vi "Registry.vi"(11 "registry actions":refnum<user-event>) -> ()   [LabVIEW 2018, in "GLog.lvlib" / "Registry.lvlib"]
uses:
  Registry.lvlib
  Registry Message.ctl
  Registry Actions.ctl
  api/logger_class/Logger.lvclass
  <vilib>/event_ctls.llb/usereventprio.ctl
  api/logger_class/Logger.lvclass/Logger.ctl
  api/Log Record.ctl
  api/logger_class/Internal Log Levels.ctl
  <vilib>/Utility/error.llb/Error Cluster From Error Code.vi
  api/logger_class/Log (Log Record).vi
  <vilib>/ErrorRing/Error Ring.xnode
  reuse_library/Utilities/Utilities.lvlib
  api/GLog.lvlib
panel:
  # "Connector Pane"
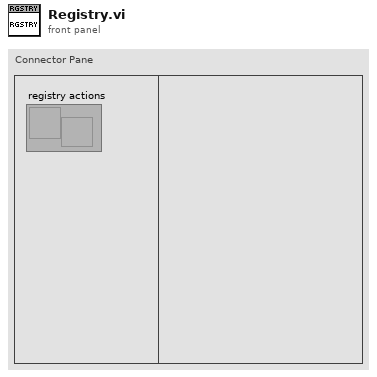
[diagram p1: front panel]
types:
  T1 = typedef "usereventprio.ctl" = enum32{"high priority", "normal priority"}
  T2 = typedef "GLog.lvlib/Registry.lvlib/Registry Message.ctl" = cluster{"action":T3, "data":variant, "return notifier":refnum<notifier>}
  T3 = typedef "GLog.lvlib/Registry.lvlib/Registry Actions.ctl" = enum16{"Register", "Log", "Enable", "Enable All", "Disable", "Disable All", "List", "Unregister", "Unregister All", "Shutdown"}
  T4 = typedef "GLog.lvlib/Log Record.ctl" = cluster{"level":T5, "timestamp":timestamp, "call chain":string[], "message":string, "data":variant}
  T5 = typedef "GLog.lvlib/Internal Log Levels.ctl" = enum16{"Trace", "Debug", "Info", "Warning", "Error", "Critical", "Internal"}
  T6 = cluster{"logger out":refnum<class "Logger.lvclass">, "empty?":bool, "error out":errorcluster}
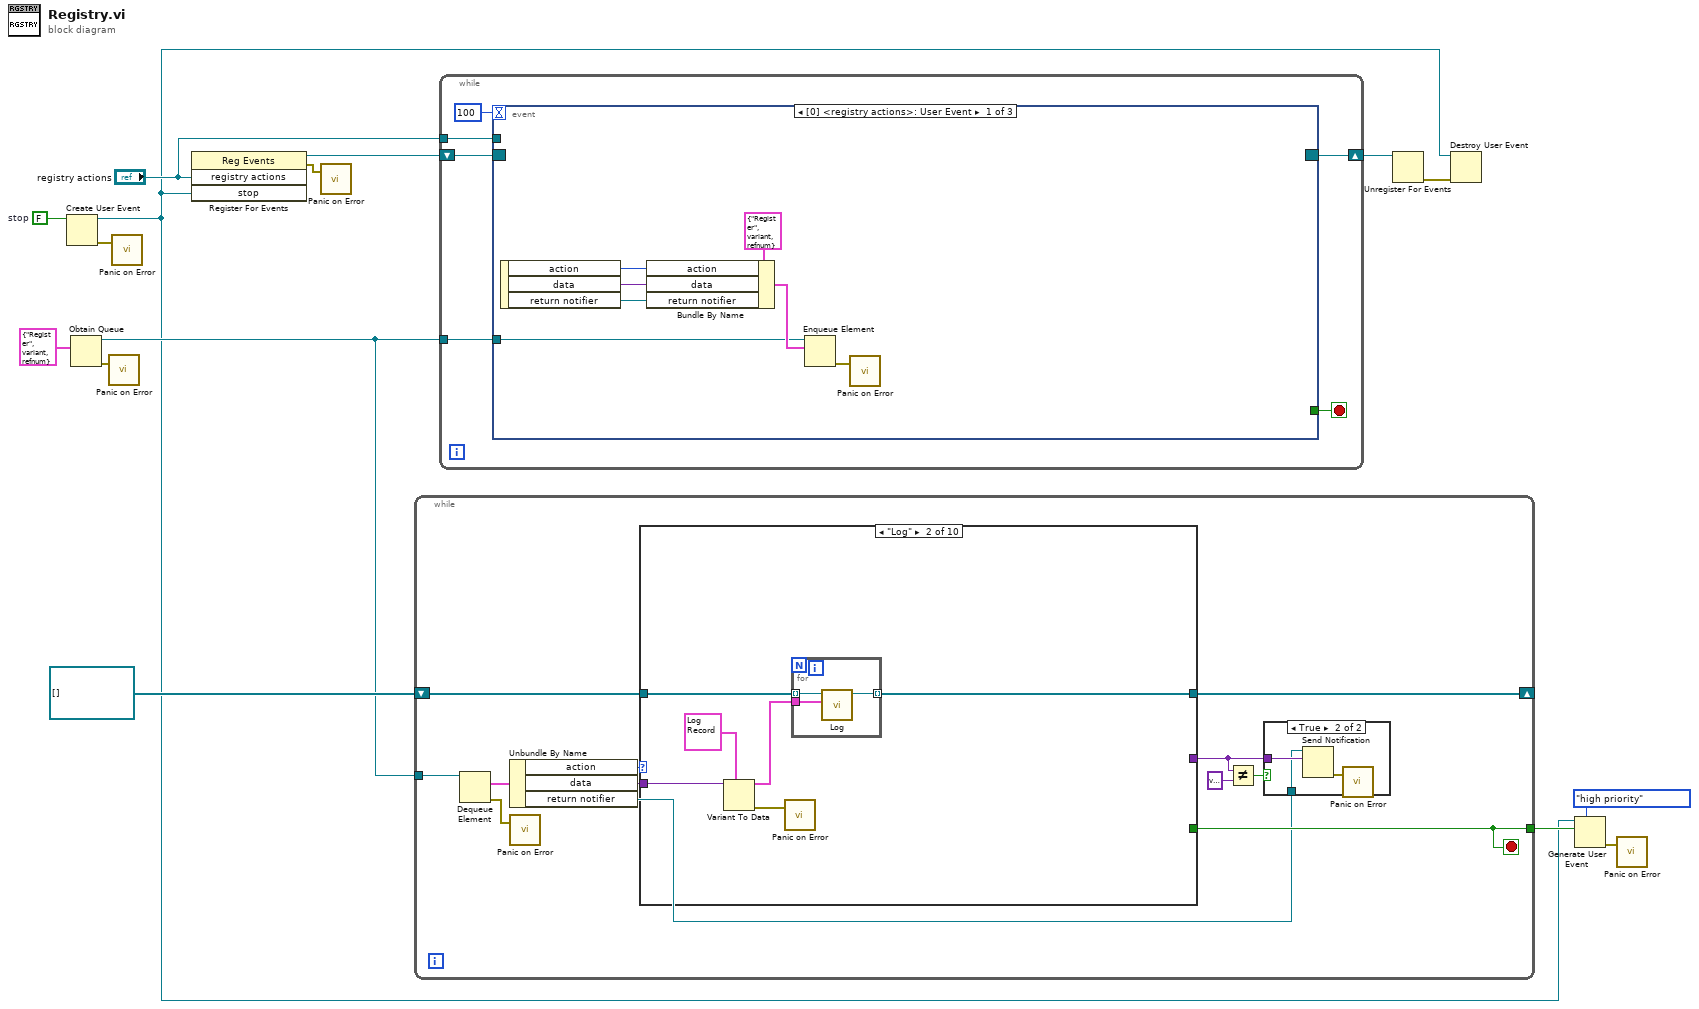
[diagram p0: block diagram]
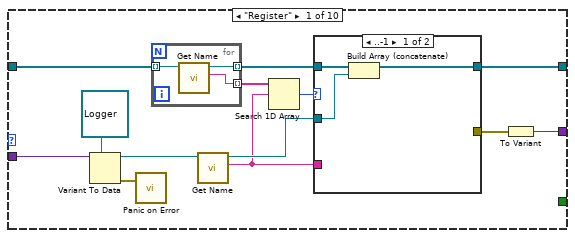
[diagram p3: hidden frame]
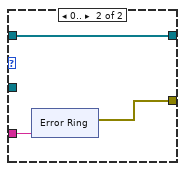
[diagram p4: hidden frame]
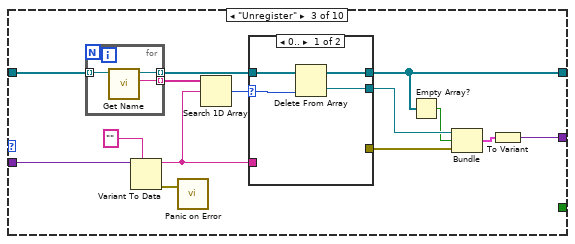
[diagram p5: hidden frame]
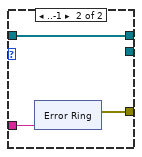
[diagram p6: hidden frame]
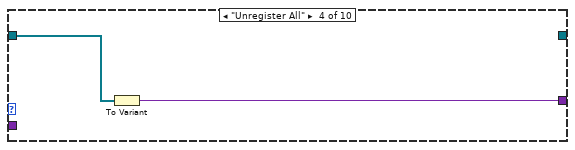
[diagram p7: hidden frame]
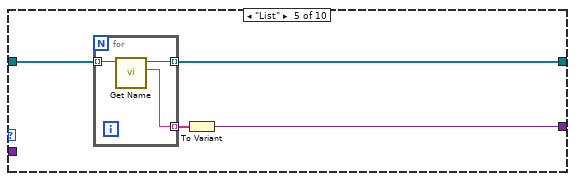
[diagram p8: hidden frame]
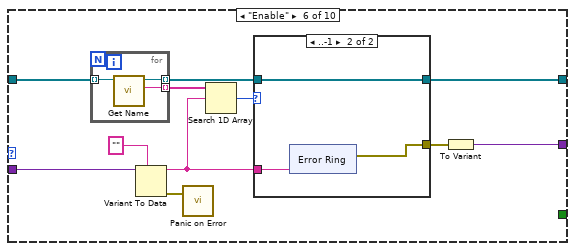
[diagram p9: hidden frame]
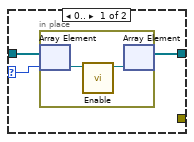
[diagram p10: hidden frame]
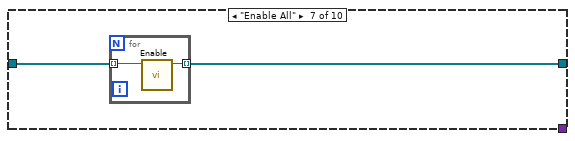
[diagram p11: hidden frame]
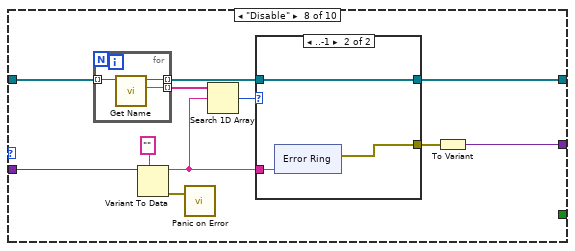
[diagram p12: hidden frame]
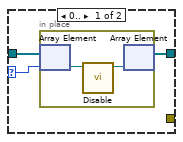
[diagram p13: hidden frame]
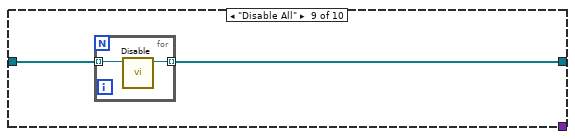
[diagram p14: hidden frame]
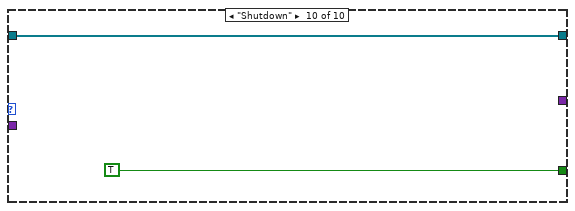
[diagram p15: hidden frame]
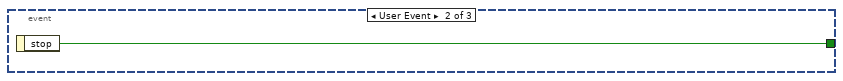
[diagram p16: hidden frame]
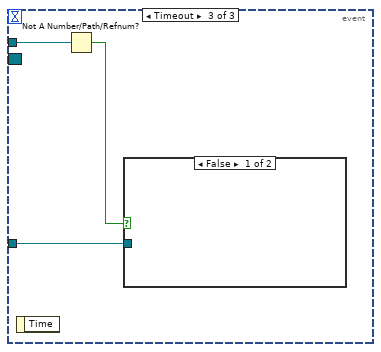
[diagram p17: hidden frame]
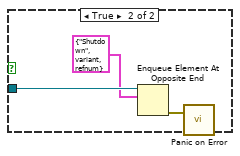
[diagram p18: hidden frame]
diagram:
  w7 = FALSE  # stop
  n1 = Create User Event(user event datatype=w7) -> (user event=w1:refnum<user-event>, error out=w6:errorcluster)  [unwired: 1 in]
  n2 = Obtain Queue(element data type=T2 {"action"=enum."Register", "data"=variant, "return notifier"=refnum} ("registry message")) -> (queue out=w13:refnum<queue>, error out=w9:errorcluster)  [unwired: 4 in, 1 out]
  n3 = call "Panic on Error.vi"("error in (no error)"=w9) -> ()  [unwired: 3 in]
  n4 = call "Panic on Error.vi"("error in (no error)"=w6) -> ()  [unwired: 3 in]
  n5 = register-events("registry actions", w1) -> (reference out=w11:refnum<event-registration>, error out=w8:errorcluster)  [unwired: 2 in]
  n6 = call "Panic on Error.vi"("error in (no error)"=w8) -> ()  [unwired: 3 in]
  n7 = while {
    shift-right: [w27] -> _
    shift-left: refnum<class "Logger.lvclass">[] [] -> [w26]
    tunnel: w13 -> [w25]
    tunnel: [w20] -> w5
    stop <- w20 stop-if-true
    n8 = Dequeue Element(queue=w25) -> (element=w23:T2, error out=w21:errorcluster)  [unwired: 2 in, 2 out]
    n9 = Unbundle By Name(w23) -> ("action"=w24:T3, "data"=w22:variant, "return notifier"=w17:refnum<notifier>)
    n10 = call "Panic on Error.vi"("error in (no error)"=w21) -> ()  [unwired: 3 in]
    n11 = case shown="\"Log\"" w24 {
      tunnel: w22 -> [w43 w64 w81 _ _ w111 _ w145 _ _]
      tunnel: [w41 w62 w70 _ w104 w112 w138 w144 w171 w176] -> w27
      tunnel: w26 -> [w39 w65 w82 w101 w105 w113 w139 w146 w172 w176]
      tunnel: [w31 _ w71 w100 w102 w109 _ w142 _ _] -> w16
      tunnel: [_ _ _ _ _ _ _ _ _ TRUE] -> w20
      frame "Register" {
        n12 = Variant To Data(type=refnum<class "Logger.lvclass"> refnum ("Logging.lvlib:Logger.lvclass"), Variant=w43) -> (data=w37:refnum<class "Logger.lvclass">, error out=w33:errorcluster)  [unwired: 1 in]
        n13 = call "Panic on Error.vi"("error in (no error)"=w33) -> ()  [unwired: 3 in]
        n14 = for {
          tunnel: w39 -> [w59] mode=indexing
          tunnel: [w58] -> w40 mode=indexing
          tunnel: [w57] -> w38 mode=indexing
          n15 = call "Get Name.vi"("logger in"=w59) -> ("name"=w57:string, "logger out"=w58:refnum<class "Logger.lvclass">)  [unwired: 9 in]
        }
        n16 = call "Get Name.vi"("logger in"=w37) -> ("name"=w34:string, "logger out"=w36:refnum<class "Logger.lvclass">)  [unwired: 9 in]
        n17 = Search 1D Array(1D array=w38, element=w34) -> (index of element=w35:i32)  [unwired: 1 in]
        n18 = case shown="..-1" w35 {
          tunnel: [w46 w49] -> w41
          tunnel: w40 -> [w45 w49]
          tunnel: w36 -> [w44 _]
          tunnel: w34 -> [_ w48]
          tunnel: [_ w47] -> w32
          frame ..-1 {
            n19 = Build Array (concatenate)(w45, w44) -> (w46:refnum<class "Logger.lvclass">[])
          }
          frame 0.. {
            n20 = xnode "Error Ring"("parameter 0"=w48) -> ("error out"=w47:errorcluster)
          }
        }
        n21 = To Variant(anything=w32) -> (Variant=w31:variant)
      }
      frame "Log" {
        n22 = Variant To Data(type=T4 {"level"=enum."Trace", "timestamp"=timestamp(0 s since 1904-01-01), "call chain"=[], "message"="", "data"=variant} ("log record"), Variant=w64) -> (data=w63:T4, error out=w61:errorcluster)  [unwired: 1 in]
        n23 = call "Panic on Error.vi"("error in (no error)"=w61) -> ()  [unwired: 3 in]
        n24 = for {
          tunnel: w65 -> [w68] mode=indexing
          tunnel: w63 -> [w66]
          tunnel: [w67] -> w62 mode=indexing
          n25 = call-poly "Log.vi"("log record"=w66, "Logger in"=w68) -> ("Logger out"=w67:refnum<class "Logger.lvclass">)  [unwired: 9 in]
        }
      }
      frame "Unregister" {
        n26 = for {
          tunnel: w82 -> [w99] mode=indexing
          tunnel: [w98] -> w79 mode=indexing
          tunnel: [w97] -> w77 mode=indexing
          n27 = call "Get Name.vi"("logger in"=w99) -> ("name"=w98:string, "logger out"=w97:refnum<class "Logger.lvclass">)  [unwired: 9 in]
        }
        n28 = Variant To Data(type="", Variant=w81) -> (data=w76:string, error out=w75:errorcluster)  [unwired: 1 in]
        n29 = call "Panic on Error.vi"("error in (no error)"=w75) -> ()  [unwired: 3 in]
        n30 = Search 1D Array(1D array=w79, element=w76) -> (index of element=w78:i32)  [unwired: 1 in]
        n31 = case shown="0.." w78 {
          selector: w78 -> [w85 _]
          tunnel: w77 -> [w86 w89]
          tunnel: [w84 w89] -> w70
          tunnel: w76 -> [_ w88]
          tunnel: [w83 _] -> w73
          tunnel: [_ w87] -> w74
          frame 0.. {
            n32 = Delete From Array(array=w86, index=w85) -> (deleted portion=w83:refnum<class "Logger.lvclass">, array with subset deleted=w84:refnum<class "Logger.lvclass">[])  [unwired: 1 in]
          }
          frame ..-1 {
            n33 = xnode "Error Ring"("parameter 0"=w88) -> ("error out"=w87:errorcluster)
          }
        }
        n34 = Empty Array?(array=w70) -> (empty?=w69:bool)
        n35 = Bundle("logger out"=w73, "empty?"=w69, "error out"=w74) -> (w72:T6)  [unwired: 1 in]
        n36 = To Variant(anything=w72) -> (Variant=w71:variant)
      }
      frame "Unregister All" {
        n37 = To Variant(anything=w101) -> (Variant=w100:variant)
      }
      frame "List" {
        n38 = for {
          tunnel: w105 -> [w108] mode=indexing
          tunnel: [w107] -> w104 mode=indexing
          tunnel: [w106] -> w103 mode=indexing
          n39 = call "Get Name.vi"("logger in"=w108) -> ("name"=w106:string, "logger out"=w107:refnum<class "Logger.lvclass">)  [unwired: 9 in]
        }
        n40 = To Variant(anything=w103) -> (Variant=w102:variant)
      }
      frame "Enable" {
        n41 = for {
          tunnel: w113 -> [w137] mode=indexing
          tunnel: [w136] -> w118 mode=indexing
          tunnel: [w135] -> w116 mode=indexing
          n42 = call "Get Name.vi"("logger in"=w137) -> ("name"=w136:string, "logger out"=w135:refnum<class "Logger.lvclass">)  [unwired: 9 in]
        }
        n43 = Variant To Data(type="", Variant=w111) -> (data=w115:string, error out=w114:errorcluster)  [unwired: 1 in]
        n44 = call "Panic on Error.vi"("error in (no error)"=w114) -> ()  [unwired: 3 in]
        n45 = Search 1D Array(1D array=w118, element=w115) -> (index of element=w117:i32)  [unwired: 1 in]
        n46 = case shown="..-1" w117 {
          selector: w117 -> [w121 _]
          tunnel: w116 -> [w122 w127]
          tunnel: [w120 w127] -> w112
          tunnel: w115 -> [_ w126]
          tunnel: [_ w125] -> w110
          frame 0.. {
            n47 = in-place {
              n48 = in-place-array #1(w122, w121) -> (w124:refnum<class "Logger.lvclass">)
              n49 = call "Enable.vi"("logger in"=w124) -> ("logger out"=w123:refnum<class "Logger.lvclass">)  [unwired: 10 in]
              n50 = in-place-array #1(w123) -> (w120:refnum<class "Logger.lvclass">[])  [unwired: 1 out]
            }
          }
          frame ..-1 {
            n51 = xnode "Error Ring"("parameter 0"=w126) -> ("error out"=w125:errorcluster)
          }
        }
        n52 = To Variant(anything=w110) -> (Variant=w109:variant)
      }
      frame "Enable All" {
        n53 = for {
          tunnel: w139 -> [w141] mode=indexing
          tunnel: [w140] -> w138 mode=indexing
          n54 = call "Enable.vi"("logger in"=w141) -> ("logger out"=w140:refnum<class "Logger.lvclass">)  [unwired: 10 in]
        }
      }
      frame "Disable" {
        n55 = for {
          tunnel: w146 -> [w170] mode=indexing
          tunnel: [w169] -> w151 mode=indexing
          tunnel: [w168] -> w149 mode=indexing
          n56 = call "Get Name.vi"("logger in"=w170) -> ("name"=w169:string, "logger out"=w168:refnum<class "Logger.lvclass">)  [unwired: 9 in]
        }
        n57 = Variant To Data(type="", Variant=w145) -> (data=w148:string, error out=w147:errorcluster)  [unwired: 1 in]
        n58 = call "Panic on Error.vi"("error in (no error)"=w147) -> ()  [unwired: 3 in]
        n59 = Search 1D Array(1D array=w151, element=w148) -> (index of element=w150:i32)  [unwired: 1 in]
        n60 = case shown="..-1" w150 {
          selector: w150 -> [w154 _]
          tunnel: w149 -> [w155 w160]
          tunnel: [w153 w160] -> w144
          tunnel: w148 -> [_ w159]
          tunnel: [_ w158] -> w143
          frame 0.. {
            n61 = in-place {
              n62 = in-place-array #2(w155, w154) -> (w157:refnum<class "Logger.lvclass">)
              n63 = call "Disable.vi"("logger in"=w157) -> ("logger out"=w156:refnum<class "Logger.lvclass">)  [unwired: 10 in]
              n64 = in-place-array #2(w156) -> (w153:refnum<class "Logger.lvclass">[])  [unwired: 1 out]
            }
          }
          frame ..-1 {
            n65 = xnode "Error Ring"("parameter 0"=w159) -> ("error out"=w158:errorcluster)
          }
        }
        n66 = To Variant(anything=w143) -> (Variant=w142:variant)
      }
      frame "Disable All" {
        n67 = for {
          tunnel: w172 -> [w174] mode=indexing
          tunnel: [w173] -> w171 mode=indexing
          n68 = call "Disable.vi"("logger in"=w174) -> ("logger out"=w173:refnum<class "Logger.lvclass">)  [unwired: 10 in]
        }
      }
      frame "Shutdown" {
      }
    }
    n69 = Not Equal?(x=w16, y=variant) -> (x != y?=w18:bool)
    n70 = case shown="True" w18 {
      tunnel: w17 -> [_ w29]
      tunnel: w16 -> [_ w30]
      frame False {
      }
      frame True {
        n71 = Send Notification(notification=w30, notifier=w29) -> (error out=w28:errorcluster)  [unwired: 1 in, 1 out]
        n72 = call "Panic on Error.vi"("error in (no error)"=w28) -> ()  [unwired: 3 in]
      }
    }
  }
  n73 = while {
    tunnel: w13 -> [w182]
    shift-right: [w180] -> w12
    shift-left: w11 -> [w179]
    tunnel: "registry actions" -> [w178]
    stop <- w177 stop-if-true
    n74 = event shown="[0] <registry actions>: User Event" {
      selector: w179 -> [_ _ _]
      dyn-events: [_ _ _] -> w180
      timeout: 100 -> [_ _ _]
      tunnel: w182 -> [w185 _ w192]
      tunnel: w178 -> [_ _ w193]
      tunnel: [_ w190 _] -> w177
      event User Event {
        n75 = event-data() -> ("action"=w188:T3, "data"=w187:variant, "return notifier"=w183:refnum<notifier>)  [unwired: 1 in]
        n76 = Bundle By Name(cluster=T2 {"action"=enum."Register", "data"=variant, "return notifier"=refnum} ("registry message"), "action"=w188, "data"=w187, "return notifier"=w183) -> (w186:T2)
        n77 = Enqueue Element(queue=w185, element=w186) -> (error out=w184:errorcluster)  [unwired: 2 in, 2 out]
        n78 = call "Panic on Error.vi"("error in (no error)"=w184) -> ()  [unwired: 3 in]
      }
      event User Event {
        n79 = event-data() -> ("stop"=w190:bool)  [unwired: 1 in]
      }
      event Timeout {
        n80 = event-data() -> ()  [unwired: 1 in, 1 out]
        n81 = Not A Number/Path/Refnum?(number/path/refnum=w193) -> (NaN/Path/Refnum?=w191:bool)
        n82 = case shown="False" w191 {
          tunnel: w192 -> [_ w196]
          frame False {
          }
          frame True {
            n83 = Enqueue Element At Opposite End(queue=w196, element=T2 {"action"=enum."Shutdown", "data"=variant, "return notifier"=refnum} ("registry message")) -> (error out=w195:errorcluster)  [unwired: 2 in, 2 out]
            n84 = call "Panic on Error.vi"("error in (no error)"=w195) -> ()  [unwired: 3 in]
          }
        }
      }
    }
  }
  n85 = Unregister For Events(event registration refnum=w12) -> (error out=w3:errorcluster)  [unwired: 1 in]
  n86 = Destroy User Event(user event=w1, error in=w3) -> ()  [unwired: 1 out]
  n87 = Generate User Event(priority (normal)=usereventprio."high priority", user event=w1, event data cluster=w5) -> (error out=w4:errorcluster)  [unwired: 1 in, 1 out]
  n88 = call "Panic on Error.vi"("error in (no error)"=w4) -> ()  [unwired: 3 in]
